vi "Report Generation.vi"(8 "error in":errorcluster, 10 "TimeStamp":string, 11 "File IO Data in":T1={"System Log File"=path "", "Data File"=path "", "Work Order Folder"=path "", "Report Template Folder"=path "", "Report Folder"=path "", "Report File"=path "", "APU Setup Folder"=path "", "Testing State"=FALSE, "Recording State"=FALSE, "Test Information"={"APU Part Number:"="", "Model:"="", "Serial Number:"="", "Customer:"="", "Work Order:"="", "Pre or Post SB"="", "Run Count"=0, "APU Selected"="<Select>"}, "Crash Log Data"=[], "Group Name"="", "APU Setup"={"Sensor Info"=[], "Variables"=[], "CMM Table 106"=[], "CMM Table 106B "=[], "Accel Config"=[], "Report Sheet 1"=[], "Report Sheet 2"=[], "Report Sheet 3"=[]}, "ChannelTagsToLog"=[], "report ref"=refnum, "APU Setup File"=path "", "RunTimes"=[], "ReportHeader"=[]} {"Test Information"."Run Count" min=0 step=1}) -> (0 "error out":errorcluster, 3 "File IO Data out":T1={"System Log File"=path "", "Data File"=path "", "Work Order Folder"=path "", "Report Template Folder"=path "", "Report Folder"=path "", "Report File"=path "", "APU Setup Folder"=path "", "Testing State"=FALSE, "Recording State"=FALSE, "Test Information"={"APU Part Number:"="", "Model:"="", "Serial Number:"="", "Customer:"="", "Work Order:"="", "Pre or Post SB"="", "Run Count"=0, "APU Selected"="<Select>"}, "Crash Log Data"=[], "Group Name"="", "APU Setup"={"Sensor Info"=[], "Variables"=[], "CMM Table 106"=[], "CMM Table 106B "=[], "Accel Config"=[], "Report Sheet 1"=[], "Report Sheet 2"=[], "Report Sheet 3"=[]}, "ChannelTagsToLog"=[], "report ref"=refnum, "APU Setup File"=path "", "RunTimes"=[], "ReportHeader"=[]} {"Test Information"."Run Count" min=0 step=1})   [LabVIEW 2018, in "File IO.lvlib"]
uses:
  File IO.lvlib
  Private Controls/File IO Data.ctl
  <vilib>/Utility/NIReport.llb/NI_report.lvclass
  Controller (Host)/Public Controls/Test Information.ctl
  Controller (Host)/Public VIs/PreorPostSB.ctl
  Controller (Host)/Public Controls/APU Select.ctl
  Top Level/Shared Controls/Analyzed Data Sets.ctl
  Top Level/Shared Controls/All Data Cluster.ctl
  Top Level/Shared Controls/Acq Data.ctl
  Top Level/Shared Controls/APU Setup File.ctl
  Public Controls/Write to Report.ctl
  Public Controls/Report Sheet Names.ctl
  <vilib>/Utility/NIReport.llb/Report Type.ctl
  Testing UI 1/Testing UI 1.lvlib
  <vilib>/Utility/NIReport.llb/NI_ReportGenerationCore.lvlib
  Controller (Host)/Controller (Host).lvlib
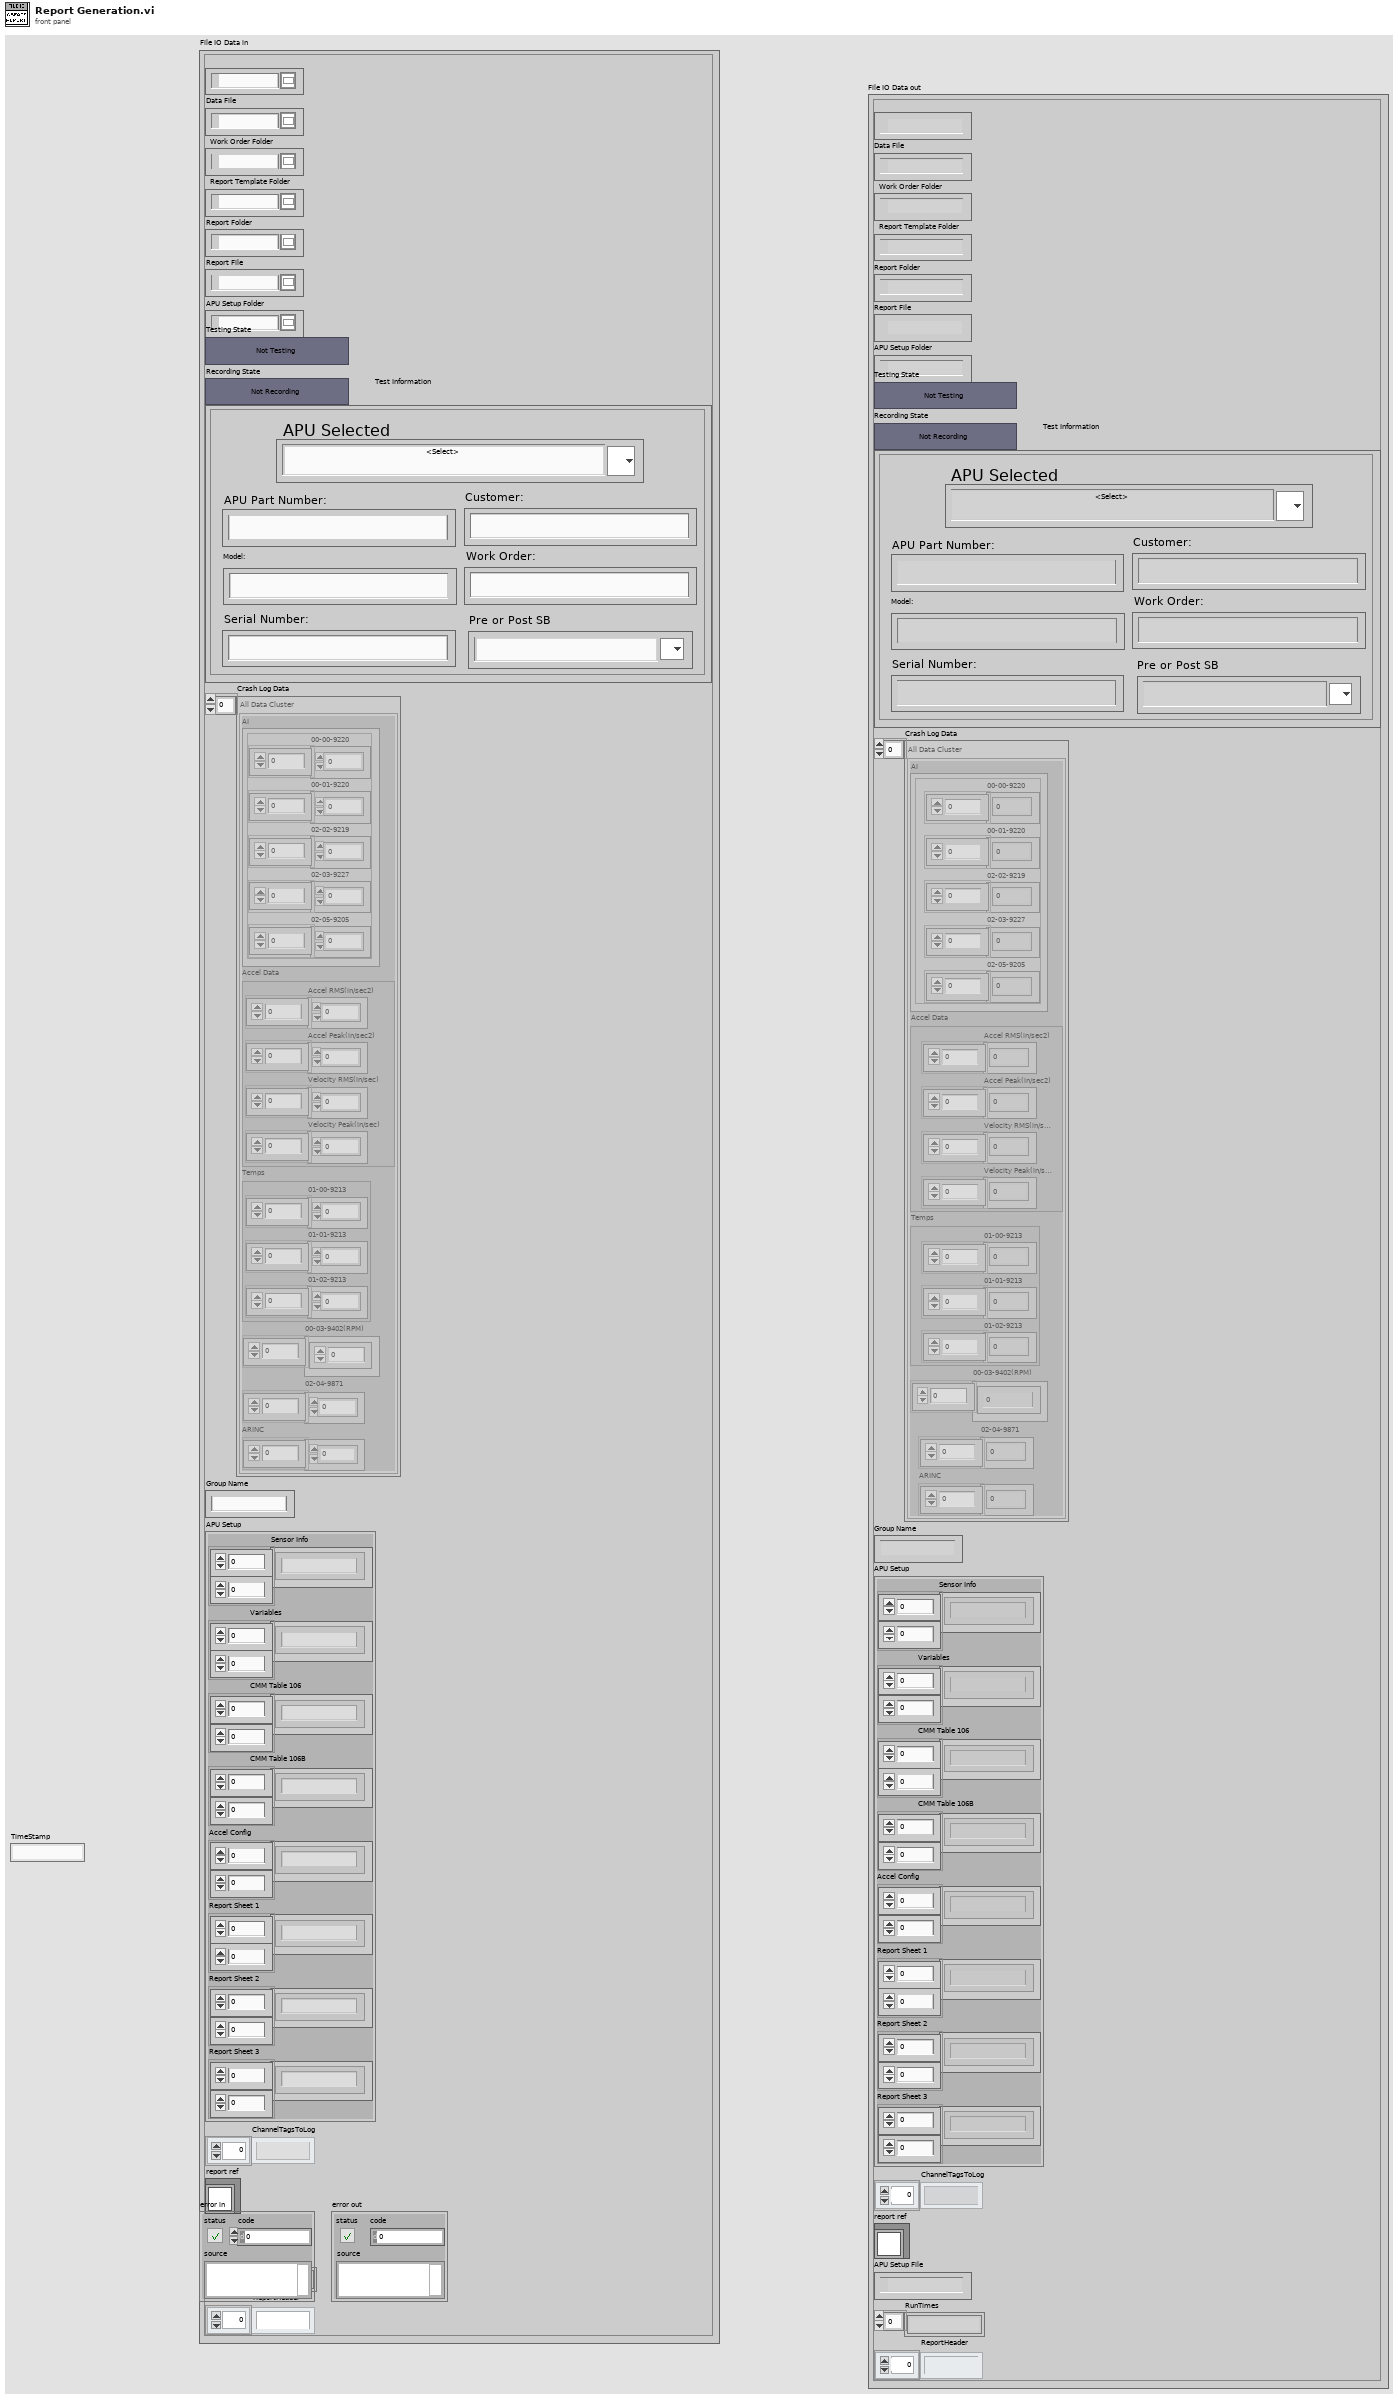
[diagram p1: front panel]
types:
  T1 = typedef "File IO.lvlib/File IO Data.ctl" = cluster{"System Log File":path, "Data File":path, "Work Order Folder":path, "Report Template Folder":path, "Report Folder":path, "Report File":path, "APU Setup Folder":path, "Testing State":bool, "Recording State":bool, "Test Information":T2, "Crash Log Data":T5, "Group Name":string, "APU Setup":T8, "ChannelTagsToLog":string[], "report ref":refnum<class "NI_report.lvclass">, "APU Setup File":path, "RunTimes":string[], "ReportHeader":string[]}
  T2 = typedef "Controller (Host).lvlib/Test Information.ctl" = cluster{"APU Part Number:":string, "Model:":string, "Serial Number:":string, "Customer:":string, "Work Order:":string, "Pre or Post SB":T3, "Run Count":i32, "APU Selected":T4}
  T3 = typedef "Controller (Host).lvlib/PreorPostSB.ctl" = string
  T4 = typedef "Controller (Host).lvlib/APU Select.ctl" = string
  T5 = typedef "Analyzed Data Sets.ctl" = T6[]
  T6 = typedef "All Data Cluster.ctl" = cluster{"AI":T7, "Accel Data":cluster{"Accel RMS(in/sec2)":dbl[], "Accel Peak(in/sec2)":dbl[], "Velocity RMS(in/sec)":dbl[], "Velocity Peak(in/sec)":dbl[]}, "Temps":cluster{"01-00-9213":dbl[], "01-01-9213":dbl[], "01-02-9213":dbl[]}, "00-03-9402(RPM)":dbl[], "02-04-9871":dbl[], "ARINC":sgl[]}
  T7 = typedef "Acq Data.ctl" = cluster{"00-00-9220":dbl[], "00-01-9220":dbl[], "02-02-9219":dbl[], "02-03-9227":dbl[], "02-05-9205":dbl[]}
  T8 = typedef "APU Setup File.ctl" = cluster{"Sensor Info":string[][], "Variables":string[][], "CMM Table 106":string[][], "CMM Table 106B ":string[][], "Accel Config":string[][], "Report Sheet 1":string[][], "Report Sheet 2":string[][], "Report Sheet 3":string[][]}
  T9 = typedef "NI_ReportGenerationCore.lvlib/Report Type.ctl" = enum16{"HTML", "Word", "Excel"}
  T10 = enum16{"maximized", "minimized", "normal", "no change"}
  T11 = typedef "File IO.lvlib/Report Sheet Names.ctl" = string
  T12 = typedef "File IO.lvlib/Write to Report.ctl" = cluster{"Sheet Name":T11, "Cell #":string, "Data":string}
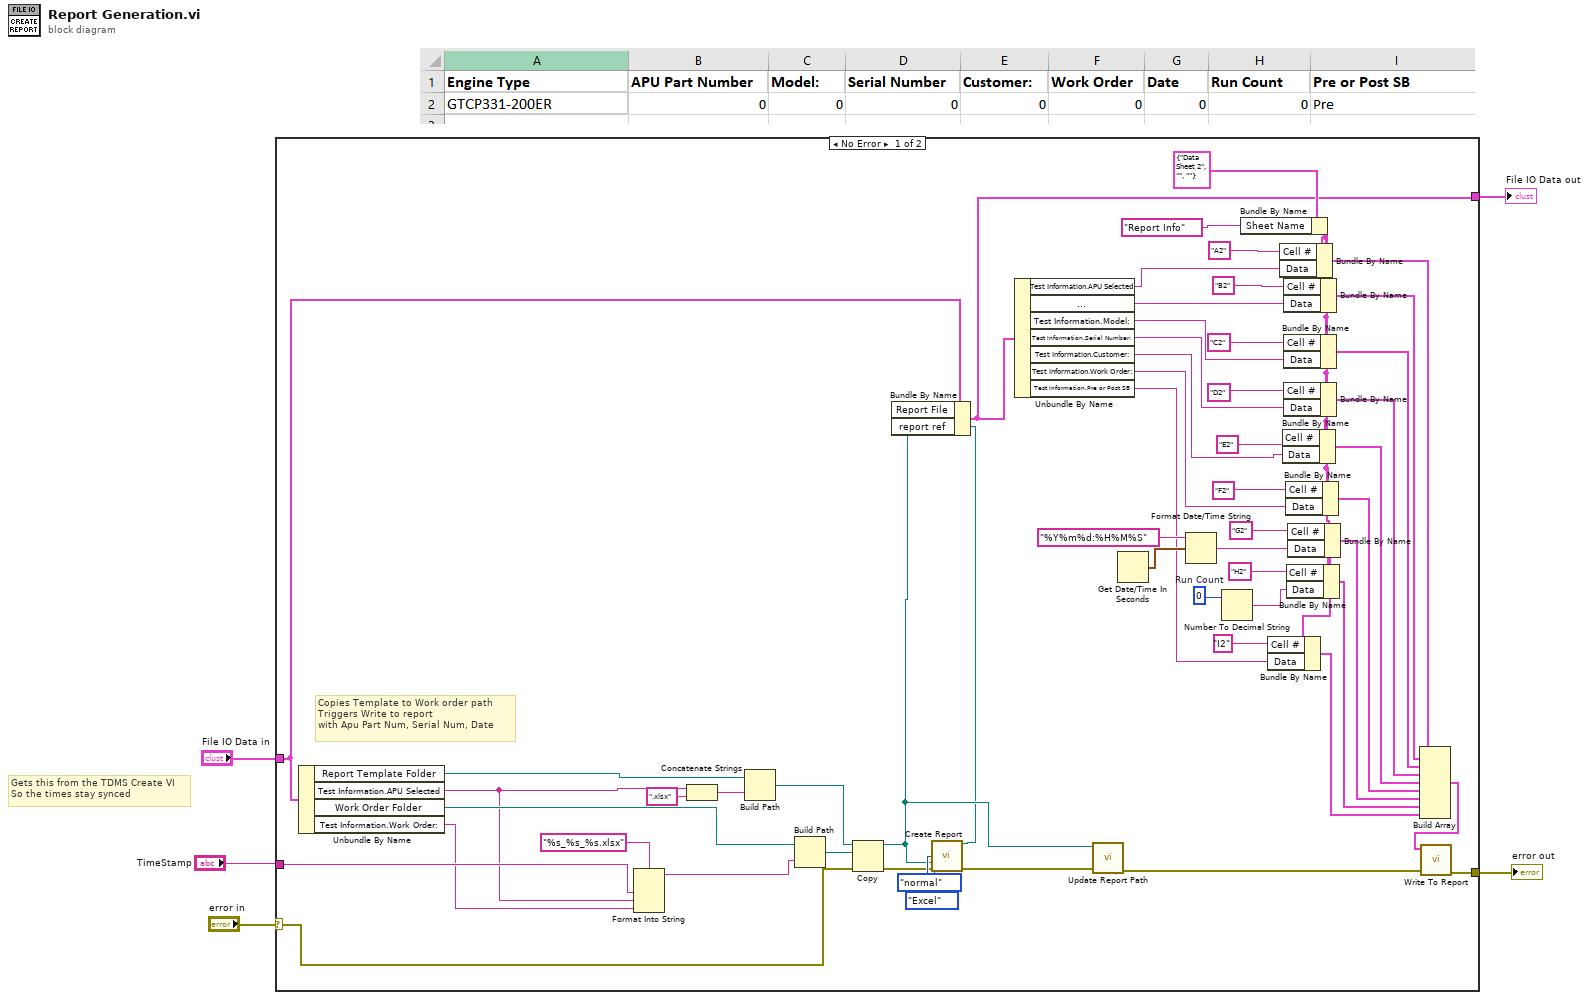
[diagram p0: block diagram]
diagram:
  # "Gets this from the TDMS Create VI\nSo the times stay synced"
  n1 = case shown="No Error" "error in" {
    selector: "error in" -> [w36 w63]
    tunnel: [w55 w63] -> w4
    tunnel: "File IO Data in" -> [w37 w62]
    tunnel: "TimeStamp" -> [w34 _]
    tunnel: [w25 w62] -> w2
    frame No Error {
      w22 = 0  # Run Count
      # "Copies Template to Work order path\nTriggers Write to report\nwith Apu Part Num, Serial Num, Date"
      n2 = Unbundle By Name(w37) -> ("Report Template Folder"=w61:path, "Test Information.APU Selected"=w30:T4, "Work Order Folder"=w59:path, "Test Information.Work Order:"=w29:string)
      n3 = Format Into String(format string="%s_%s_%s.xlsx", w34, w30, w29) -> (resulting string=w33:string)  [unwired: 2 in, 1 out]
      n4 = Concatenate Strings(w30, ".xlsx" ("string")) -> (w31:string)
      n5 = Build Path(base path=w61, name or relative path=w31) -> (appended path=w60:path)
      n6 = Build Path(base path=w59, name or relative path=w33) -> (appended path=w58:path)
      n7 = Copy(8:w36, 10:w58, 11:w60) -> (0:w10:errorcluster, 3:w8:path)  [unwired: 2 in, 1 out]
      n8 = call <vilib>:"Create Report.vi"("window state (normal)"=T10."normal", "report type"=Report_Type."Excel", "template (empty)"=w8, "error in (no error)"=w10) -> ("report out"=w7:refnum<class "NI_report.lvclass">, "error out"=w9:errorcluster)  [unwired: 10 in]
      n9 = Bundle By Name(cluster=w37, "Report File"=w8, "report ref"=w7) -> (w25:T1)
      n10 = Unbundle By Name(w25) -> ("Test Information.APU Selected"=w14:T4, "Test Information.APU Part Number:"=w45:string, "Test Information.Model:"=w44:string, "Test Information.Serial Number:"=w43:string, "Test Information.Customer:"=w42:string, "Test Information.Work Order:"=w6:string, "Test Information.Pre or Post SB"=w18:T3)
      n11 = call "Update Report Path.vi"("error in (no error)"=w9, "Report Path"=w8) -> ("error out"=w24:errorcluster)  [unwired: 9 in]
      n12 = Get Date/Time In Seconds() -> (seconds since 1Jan1904=w57:timestamp)
      n13 = Format Date/Time String(time format string (%c)="%Y%m%d:%H%M%S", seconds (now)=w57) -> (date/time string=w41:string)  [unwired: 1 in]
      n14 = Number To Decimal String(number=w22) -> (decimal integer string=w21:string)  [unwired: 1 in]
      n15 = Bundle By Name(cluster=T12 {"Sheet Name"="Data Sheet 2", "Cell #"="", "Data"=""}, "Sheet Name"=T11 "Report Info") -> (w15:T12)
      n16 = Bundle By Name(cluster=w15, "Cell #"="I2", "Data"=w18) -> (w17:T12)
      n17 = Bundle By Name(cluster=w15, "Cell #"="A2", "Data"=w14) -> (w13:T12)
      n18 = Bundle By Name(cluster=w15, "Cell #"="E2", "Data"=w42) -> (w40:T12)
      n19 = Bundle By Name(cluster=w15, "Cell #"="B2", "Data"=w45) -> (w51:T12)
      n20 = Bundle By Name(cluster=w15, "Cell #"="C2", "Data"=w44) -> (w50:T12)
      n21 = Bundle By Name(cluster=w15, "Cell #"="D2", "Data"=w43) -> (w49:T12)
      n22 = Bundle By Name(cluster=w15, "Cell #"="F2", "Data"=w6) -> (w39:T12)
      n23 = Bundle By Name(cluster=w15, "Cell #"="H2", "Data"=w21) -> (w20:T12)
      n24 = Bundle By Name(cluster=w15, "Cell #"="G2", "Data"=w41) -> (w38:T12)
      n25 = Build Array(w13, w51, w50, w49, w40, w39, w38, w20, w17) -> (w28:T12[])
      n26 = call "Write To Report.vi"("error in (no error)"=w24, "Report Info"=w28) -> ("error out"=w55:errorcluster)  [unwired: 9 in]
    }
    frame Error {
      # "Propogate Error through subvi"
    }
  }
  "error out" <- w4
  "File IO Data out" <- w2
